vi "set minimum FPS.vi"(8 "error in (no error)":errorcluster, 11 "Thorcam in":refnum<class "Thorcam.lvclass">) -> (0 "error out":errorcluster, 3 "Thorcam out":refnum<class "Thorcam.lvclass">)   [LabVIEW 2012, in "Thorcam.lvclass"]
uses:
  Thorcam.lvclass
  Thorcam.lvclass/Thorcam.ctl
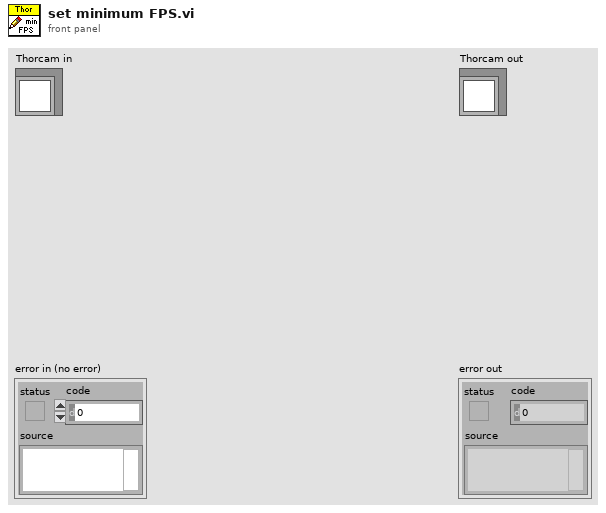
[diagram p1: front panel]
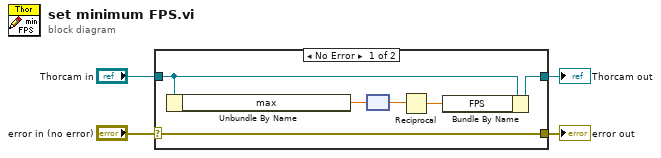
[diagram p0: block diagram]
diagram:
  n1 = case shown="No Error" "error in (no error)" {
    selector: "error in (no error)" -> [w10 w12]
    tunnel: [w10 w12] -> w3
    tunnel: [w6 w11] -> w1
    tunnel: "Thorcam in" -> [w7 w11]
    frame No Error {
      n2 = Unbundle By Name(w7) -> ("max"=w8:dbl[unit])
      n3 = node(w8) -> (w9:dbl)
      n4 = Reciprocal(x=w9) -> (1/x=w5:dbl)
      n5 = Bundle By Name(cluster=w7, "FPS"=w5) -> (w6:refnum<class "Thorcam.lvclass">)
    }
    frame Error {
    }
  }
  "error out" <- w3
  "Thorcam out" <- w1
